vi "Library Resolve VI Path.vi"(5 "VI name":string, 11 "sub path of toolkit (none)":path) -> (6 "VI path":path)   [LabVIEW 2012]
doc: "Takes the name of a VI and an optional toolkit subpath and resolves its location for the current runtime in a manner that works when built and when running in development mode. In development mode, the VI is assumed to be located in the directory of the toolkit/library/class as can be extracted from the VI name. When built, the VI is assumed to be located in the application executable unless evidence is found that VIs are located inside a source tree located outside the executable. The latter case might occur when a minimal executable is built that loads VIs dynamically from the development source tree."
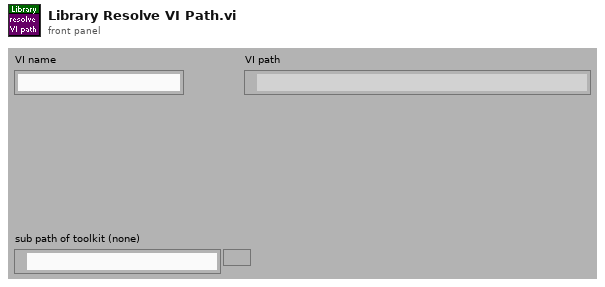
[diagram p1: front panel]
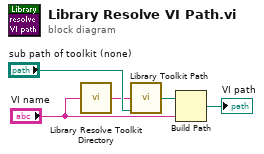
[diagram p0: block diagram]
diagram:
  n1 = call "Library Resolve Toolkit Directory.vi"("VI name"="VI name") -> ("toolkit directory"=w2:string)
  n2 = call "Library Toolkit Path.vi"("toolkit directory (none)"=w2, "sub path of toolkit (none)"="sub path of toolkit (none)") -> ("absolute toolkit path"=w4:path)  [unwired: 13 in]
  n3 = Build Path(base path=w4, name or relative path="VI name") -> (appended path=→"VI path":path)
